vi "Receiver_Example.vi"() -> ()   [LabVIEW 2022 SP3]
panel:
  in  "Decode SC?":bool
  out "created new?":bool
  out "XY Graph":cdb[](graph)
  out "Modulation parameter":T1
  out "string 2":string
  out "SIG valid?":bool
  out "Frequency offset":dbl
  in  "stop":bool
  out "USRP CoercedParamters":T2={"coerced IQ rate"=100000.0, "coerced carrier frequency"=100000.0, "coerced gain"=0.0} {"coerced gain" format="%#_6f"; "coerced carrier frequency" format="%#_6p"; "coerced IQ rate" format="%#_6p"}
  out "error out":errorcluster
  in  "Trigger level":dbl=0.005 format="%f"
  in  "error in (no error)":errorcluster
  in  "USRP ControledParameters":T3={"active antenna"="RX2", "gain"=3.0, "carrier frequency"=2400000000.0, "IQ rate"=2000000.0} {"IQ rate" format="%#_6p"; "carrier frequency" format="%#_6p"; "gain" format="%#_6f"}
  in  "device names":refnum<k15>="RIO0"
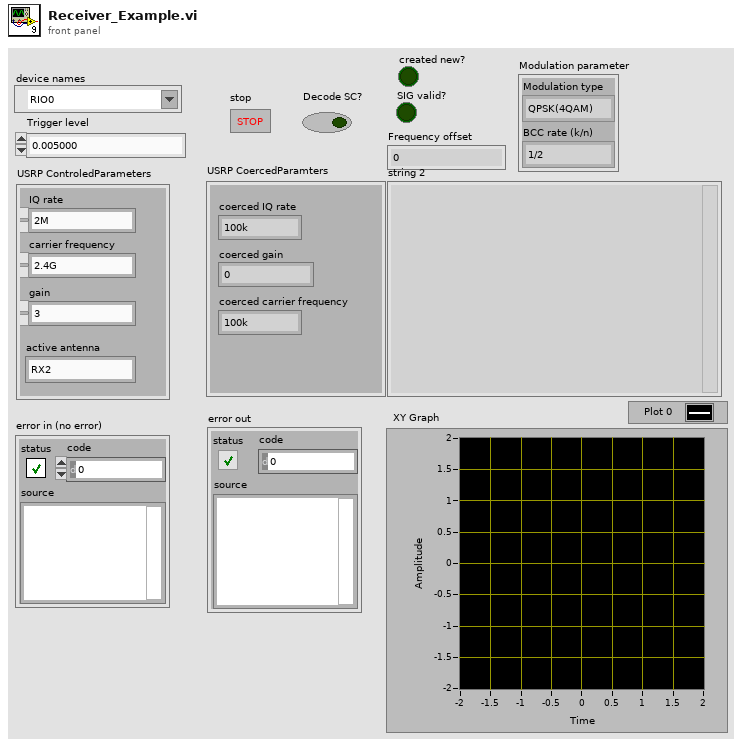
[diagram p1: front panel]
types:
  T1 = cluster{"Modulation type":enum16{"QPSK(4QAM)", "64QAM", "16QAM", "BPSK"}, "BCC rate (k/n)":enum16{"1/2", "2/3", "3/4"}}
  T2 = cluster{"coerced IQ rate":dbl, "coerced carrier frequency":dbl, "coerced gain":dbl}
  T3 = cluster{"active antenna":string, "gain":dbl, "carrier frequency":dbl, "IQ rate":dbl}
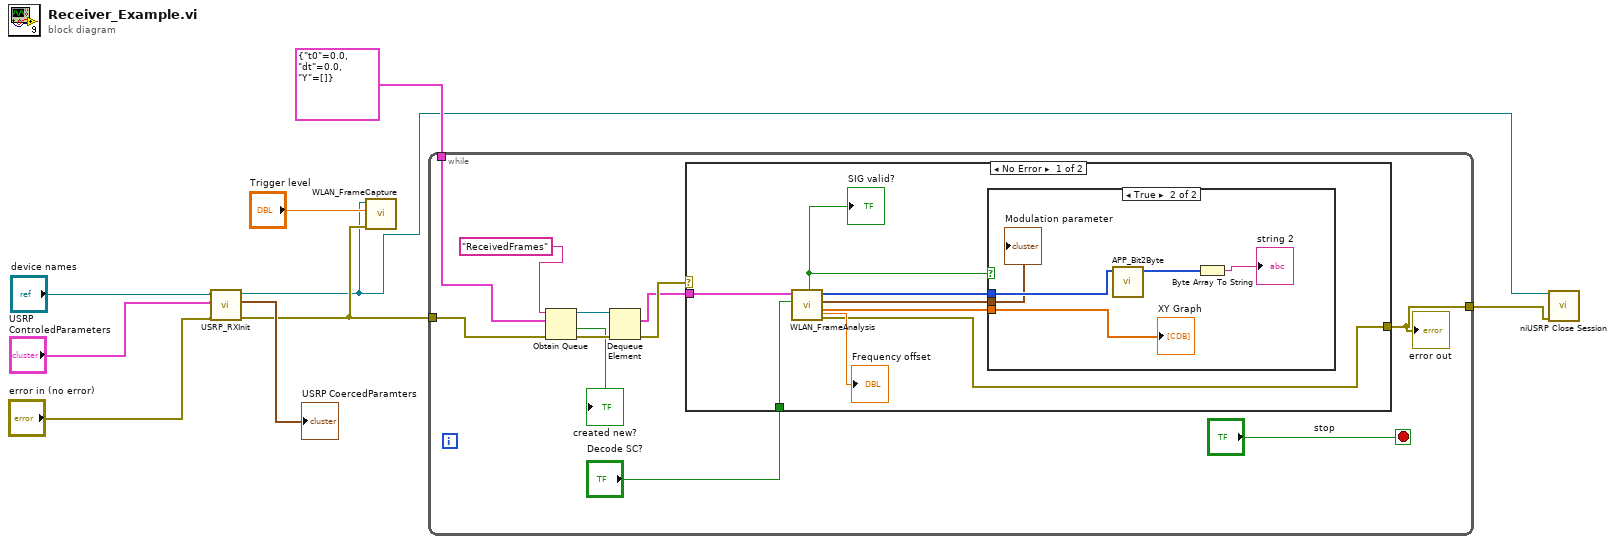
[diagram p0: block diagram]
diagram:
  n1 = call "USRP_RXInit.vi"("device names"="device names", "USRP ControledParameters"="USRP ControledParameters", "error in (no error)"="error in (no error)") -> ("session handle out"=w1:refnum<k15>, "USRP CoercedParamters"=→"USRP CoercedParamters":T2, "error out"=w5:errorcluster)  [unwired: 5 in]
  n2 = call "WLAN_FrameCapture.vi"("error in (no error)"=w5, "Trigger level"="Trigger level", "session handle"=w1) -> ()  [unwired: 8 in]
  n3 = while {
    tunnel: w5 -> [w18]
    tunnel: cluster{"t0":dbl, "dt":dbl, "Y":cdb[]} {"t0"=0.0, "dt"=0.0, "Y"=[]} ("data") -> [w19]
    tunnel: [w11] -> w2
    stop <- "stop" stop-if-true
    n4 = Obtain Queue(name (unnamed)="ReceivedFrames", element data type=w19, error in (no error)=w18) -> (queue out=w17:refnum<queue>, created new?=→"created new?":bool, error out=w14:errorcluster)  [unwired: 2 in]
    n5 = Dequeue Element(queue=w17, error in (no error)=w14) -> (element=w15:cluster{"t0":dbl, "dt":dbl, "Y":cdb[]}, error out=w16:errorcluster)  [unwired: 1 in, 2 out]
    n6 = case shown="No Error" w16 {
      selector: w16 -> [_ w34]
      tunnel: w15 -> [w22 _]
      tunnel: [w23 w34] -> w11
      tunnel: "Decode SC?" -> [w21 _]
      frame No Error {
        n7 = call "WLAN_FrameAnalysis.vi"("Decode SC"=w21, "input cluster"=w22) -> ("error out"=w23:errorcluster, "Constellation"=w25:cdb[], "Modulation parameter"=w24:T1, "output bits"=w26:i8[], "Frequency offset"=→"Frequency offset":dbl, "SIG valid?"=w27:bool)  [unwired: 4 in]
        "SIG valid?" <- w27
        n8 = case shown="True" w27 {
          tunnel: w26 -> [_ w33]
          tunnel: w25 -> [_ w31]
          tunnel: w24 -> [_ w32]
          frame False {
          }
          frame True {
            n9 = call "APP_Bit2Byte.vi"("input bit stream"=w33) -> ("output byte stream"=w29:u8[])  [unwired: 10 in]
            n10 = Byte Array To String(unsigned byte array=w29) -> (string=→"string 2":string)
            "Modulation parameter" <- w32
            "XY Graph" <- w31
          }
        }
      }
      frame Error {
      }
    }
    "error out" <- w11
  }
  n11 = call <instrlib>:"niUSRP Close Session.vi"("session handle"=w1, "error in (no error)"=w2) -> ()  [unwired: 13 in, 1 out]
